vi "Fetch - DBL.vi"(7 "PV name":string, 8 "error in":errorcluster, 10 "default":dbl, 11 "Server in":refnum<class "Server.lvclass">) -> (0 "error out":errorcluster, 1 "PV not found?":bool, 2 "value":dbl, 3 "Server out":refnum<class "Server.lvclass">, 4 "timestamp":timestamp)   [LabVIEW 2020, in "PV Access.lvlib" / "PVA Server.lvlib" / "Server.lvclass"]
uses:
  Server.lvclass
  Server.lvclass/Server.ctl
  c7e3d648-f322-44e9-8ea0-79ff1b27e4c3.vi
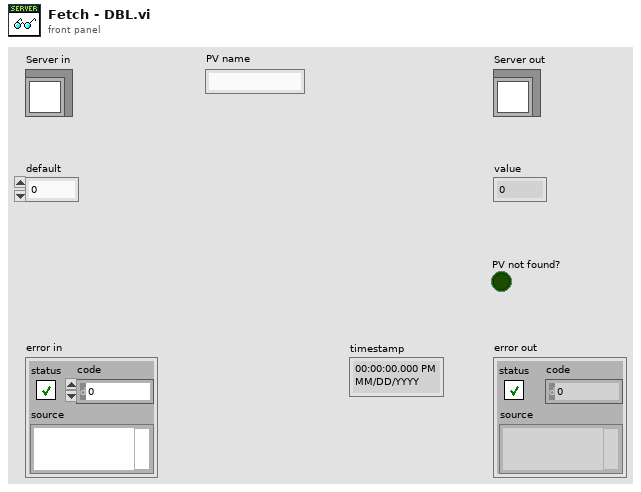
[diagram p1: front panel]
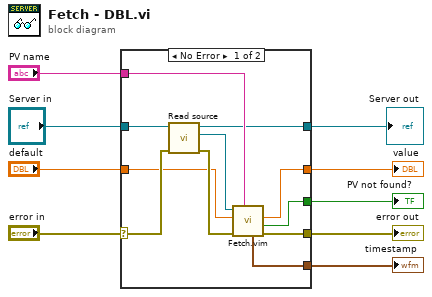
[diagram p0: block diagram]
diagram:
  n1 = case shown="No Error" "error in" {
    selector: "error in" -> [w18 w21]
    tunnel: [w20 w21] -> w9
    tunnel: "PV name" -> [w19 _]
    tunnel: [w17 _] -> w6
    tunnel: "Server in" -> [w15 w23]
    tunnel: [w14 w23] -> w4
    tunnel: "default" -> [w12 w22]
    tunnel: [w11 w22] -> w2
    tunnel: [w10 _] -> w1
    frame No Error {
      n2 = call "Read source.vi"("error in (no error)"=w18, "Server in"=w15) -> ("error out"=w16:errorcluster, "Source"=w13:refnum<class "Source.lvclass">, "Server out"=w14:refnum<class "Server.lvclass">)  [unwired: 7 in]
      n3 = call "Fetch.vim"("PV name"=w19, "error in"=w16, "data type"=w12, "Source in"=w13) -> ("error out"=w20:errorcluster, "PV not found?"=w10:bool, "value"=w11:dbl, "timestamp"=w17:timestamp)  [unwired: 3 in, 1 out]
    }
    frame Error {
    }
  }
  "Server out" <- w4
  "error out" <- w9
  "timestamp" <- w6
  "value" <- w2
  "PV not found?" <- w1
